vi "Solve PnP (IPPESquare).vi"(6 "Camera Parameters":T6, 7 "Square Length":dbl, 8 "error in (no error)":errorcluster, 11 "Square Corners":T1) -> (0 "error out":errorcluster, 3 "Pose":T3)   [LabVIEW 2020, in "g_ar_toolkit.ar.lvlib"]
uses:
  g_ar_toolkit.ar.lvlib
  g_ar_toolkit.common/Camera Parameters.ctl
  g_ar_toolkit.common/Camera Matrix.ctl
  g_ar_toolkit.common/Camera Distortion Coefficients.ctl
  Pose.ctl
  rvec.ctl
  g_ar_toolkit.common/tvec.ctl
  g_ar_toolkit.common/Square Corners.ctl
  g_ar_toolkit.common/Image Point (Float).ctl
  Point Correspondence Set.ctl
  g_ar_toolkit.common/Object Point (Float).ctl
  SolvePnPFlags.ctl
  g_ar_toolkit.common/Module Path.vi
  <vilib>/Utility/error.llb/Error Cluster From Error Code.vi
  g_ar_toolkit.common/g_ar_toolkit.common.lvlib
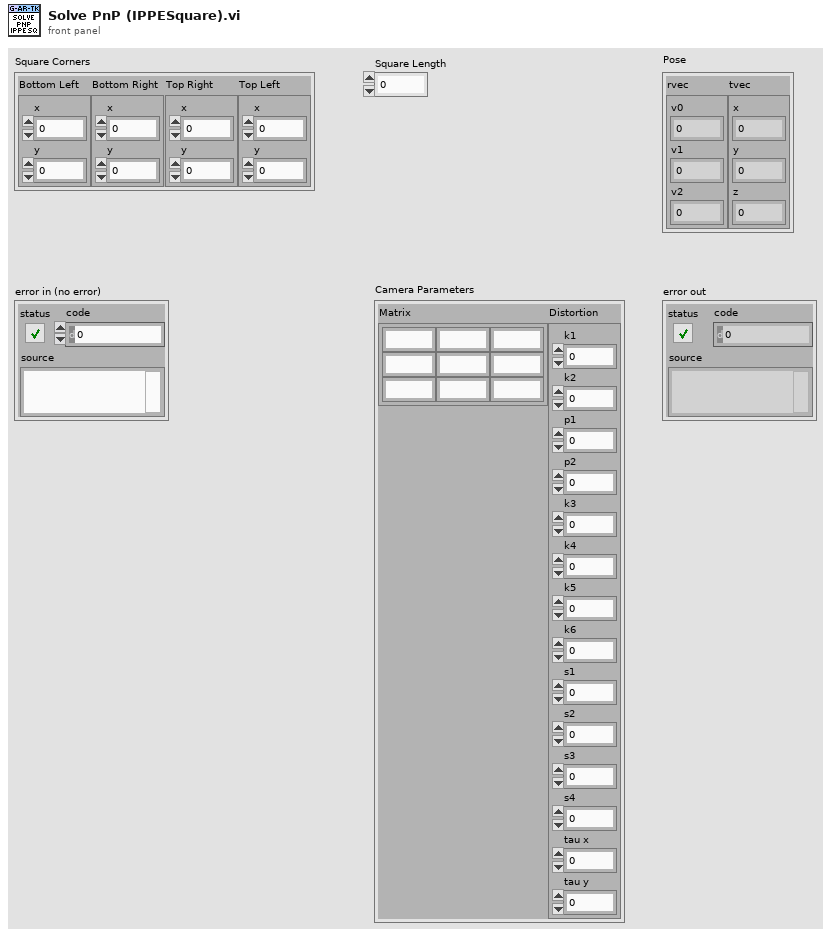
[diagram p1: front panel]
types:
  T1 = typedef "g_ar_toolkit.common.lvlib/Square Corners.ctl" = cluster{"Bottom Left":T2, "Bottom Right":T2, "Top Right":T2, "Top Left":T2}
  T2 = typedef "g_ar_toolkit.common.lvlib/Image Point (Float).ctl" = cluster{"x":dbl, "y":dbl}
  T3 = typedef "g_ar_toolkit.ar.lvlib/Pose.ctl" = cluster{"rvec":T4, "tvec":T5}
  T4 = typedef "g_ar_toolkit.ar.lvlib/rvec.ctl" = cluster{"v0":dbl, "v1":dbl, "v2":dbl}
  T5 = typedef "g_ar_toolkit.ar.lvlib/tvec.ctl" = cluster{"x":dbl, "y":dbl, "z":dbl}
  T6 = typedef "g_ar_toolkit.common.lvlib/Camera Parameters.ctl" = cluster{"Matrix":T7, "Distortion":T8}
  T7 = typedef "g_ar_toolkit.common.lvlib/Camera Matrix.ctl" = cluster{"m 0,0":dbl, "m 0,1":dbl, "m 0,2":dbl, "m 1,0":dbl, "m 1,1":dbl, "m 1,2":dbl, "m 2,0":dbl, "m 2,1":dbl, "m 2,2":dbl}
  T8 = typedef "g_ar_toolkit.common.lvlib/Camera Distortion Coefficients.ctl" = cluster{"k1":dbl, "k2":dbl, "p1":dbl, "p2":dbl, "k3":dbl, "k4":dbl, "k5":dbl, "k6":dbl, "s1":dbl, "s2":dbl, "s3":dbl, "s4":dbl, "tau x":dbl, "tau y":dbl}
  T9 = typedef "g_ar_toolkit.ar.lvlib/Point Correspondence Set.ctl" = cluster{"Object Points":T10[], "Image Points":T2[]}
  T10 = typedef "g_ar_toolkit.common.lvlib/Object Point (Float).ctl" = cluster{"x":dbl, "y":dbl, "z":dbl}
  T11 = typedef "g_ar_toolkit.ar.lvlib/SolvePnPFlags.ctl" = enum8{"SOLVEPNP_ITERATIVE", "SOLVEPNP_EPNP", "SOLVEPNP_P3P", "SOLVEPNP_AP3P", "SOLVEPNP_IPPE", "SOLVEPNP_IPPE_SQUARE", "SOLVEPNP_SQPNP"}
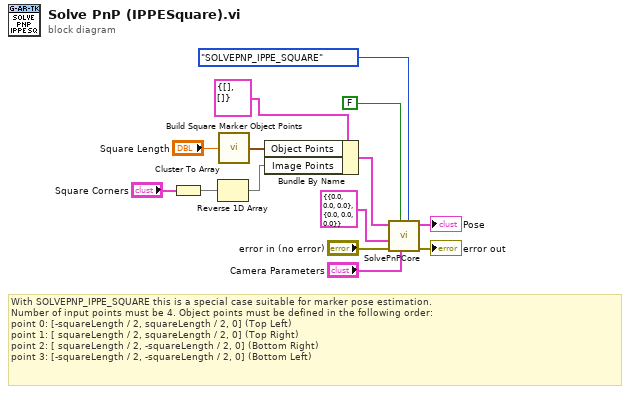
[diagram p0: block diagram]
diagram:
  # "With SOLVEPNP_IPPE_SQUARE this is a special case suitable for marker pose estimation. \nNumber of input points must be 4. Object points must be defined in the following order:\npoint 0: [-squareLength / 2, squareLength / 2, 0] (Top Left)\npoint 1: [ squareLength / 2, squareLength / 2, 0] (Top Right)\npoint 2: [ squareLength / 2, -squareLength / 2, 0] (Bottom Right)\npoint 3: [-squareLength / 2, -squareLength / 2, 0] (Bottom Left)"
  n1 = Cluster To Array(cluster="Square Corners") -> (array=w12:T2[])
  n2 = Reverse 1D Array(array=w12) -> (reversed array=w2:T2[])
  n3 = call "Build Square Marker Object Points.vi"("Square Length"="Square Length") -> ("Points"=w3:T10[])
  n4 = Bundle By Name(cluster=T9 {"Object Points"=[], "Image Points"=[]} ("Point Correspondence Set"), "Object Points"=w3, "Image Points"=w2) -> (w4:T9)
  n5 = call "SolvePnPCore.vi"("Solve PnP Flags"=SolvePnPFlags."SOLVEPNP_IPPE_SQUARE", "Camera Parameters"="Camera Parameters", "Use Pose Guess"=FALSE ("Use Iterative"), "error in (no error)"="error in (no error)", "Pose (Estimate) in"=T3 {"rvec"={"v0"=0.0, "v1"=0.0, "v2"=0.0}, "tvec"={"x"=0.0, "y"=0.0, "z"=0.0}} ("Pose (Estimate)"), "Point Correspondence Set"=w4) -> ("error out"=→"error out":errorcluster, "Pose"=→"Pose":T3)  [unwired: 4 in]
